vi "Workspace - Save.vi"(7 "_Subhost-FP.DockStates":bool[](array[boolean]), 8 "error in":errorcluster, 9 "This VI":refnum<vi>, 10 "VI Refs":refnum<vi>[](array[refnum]), 11 "Subhost Names":string[](array[string])) -> (0 "error out":errorcluster, 2 "VI Refs out":refnum<vi>[](array[refnum]), 3 "Subhost Names out":string[](array[string]))   [LabVIEW 2016]
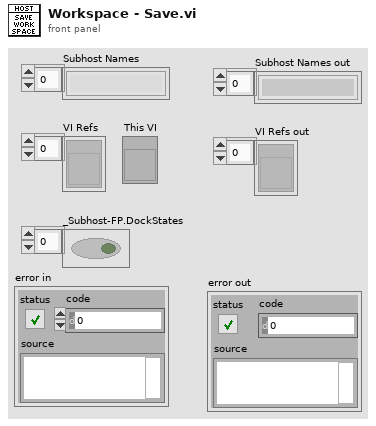
[diagram p1: front panel]
types:
  T1 = enum16{"open", "replace", "create", "open or create", "replace or create", "replace or create with confirmation"}
  T2 = typedef "LVRectTypeDef.ctl" = cluster{"Left":i16, "Top":i16, "Right":i16, "Bottom":i16}
  T3 = enum32{"Invalid", "Standard", "Closed", "Hidden", "Minimized", "Maximized"}
  T4 = cluster{"Display Name":string, "Front Panel.WinBounds":T2, "FP.State":enum32{"Invalid", "Standard", "Closed", "Hidden", "Minimized", "Maximized"}, "FP.Monitor":u16, "Boolean":bool}
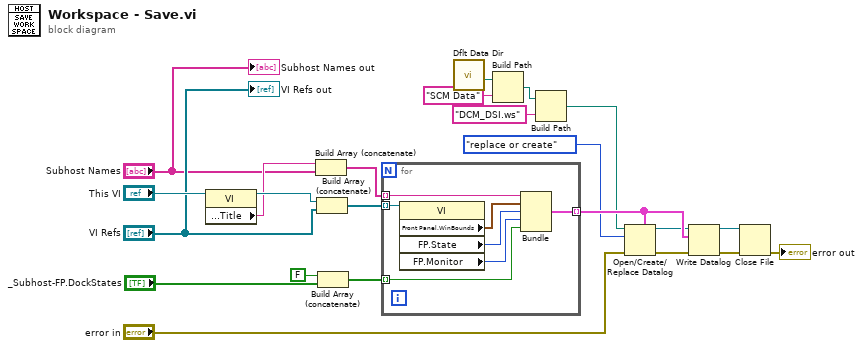
[diagram p0: block diagram]
diagram:
  n1 = property class="VI"(reference="This VI") -> (reference out=w12:refnum<vi>, "Front Panel.Title"=w11:string)  [unwired: 1 in, 1 out]
  n2 = Build Array (concatenate)(w11, "Subhost Names") -> (w13:string[])
  n3 = Build Array (concatenate)(w12, "VI Refs") -> (w15:refnum<vi>[])
  n4 = Build Array (concatenate)(FALSE ("Boolean"), "_Subhost-FP.DockStates") -> (w9:bool[])
  n5 = for {
    tunnel: w15 -> [w30] mode=indexing
    tunnel: w9 -> [w26] mode=indexing
    tunnel: w13 -> [w27] mode=indexing
    tunnel: [w25] -> w20 mode=indexing
    n6 = property class="VI"(reference=w30) -> ("Front Panel.WinBounds"=w28:T2, "FP.State"=w29:T3, "FP.Monitor"=w24:u16)  [unwired: 1 in, 2 out]
    n7 = Bundle("Display Name"=w27, "Front Panel.WinBounds"=w28, "FP.State"=w29, "FP.Monitor"=w24, "Boolean"=w26) -> (w25:T4)  [unwired: 1 in]
  }
  n8 = call <vilib>:"Dflt Data Dir.vi"() -> ("App:Default Data Directory"=w3:path)
  n9 = Build Path(base path=w3, name or relative path="SCM Data") -> (appended path=w1:path)
  n10 = Build Path(base path=w1, name or relative path="DCM_DSI.ws") -> (appended path=w17:path)
  n11 = Open/Create/Replace Datalog(5:w20, 8:"error in", 10:T1."replace or create" ("operation (0:open)"), 11:w17) -> (0:w21:errorcluster, 3:w19:refnum<k1>)  [unwired: 2 in, 1 out]
  n12 = Write Datalog(4:w21, 6:w20, 7:w19) -> (0:w23:errorcluster, 3:w22:refnum<k1>)
  n13 = Close File(refnum=w22, error in=w23) -> (error out=→"error out":errorcluster)  [unwired: 1 out]
  "Subhost Names out" <- "Subhost Names"
  "VI Refs out" <- "VI Refs"
